vi "Launch Event Handlers.vi"(8 "error in (no error)":errorcluster, 11 "IViewable In":refnum<class "IViewable.lvclass">) -> (0 "error out":errorcluster, 3 "IViewable Out":refnum<class "IViewable.lvclass">)   [LabVIEW 2020, in "MVA Framework.lvlib" / "IViewable.lvlib" / "IViewable.lvclass"]
doc: "启动事件处理程序"
uses:
  IViewable.lvclass
  ActorEvents/IEventAggregator/IEventAggregator.lvclass
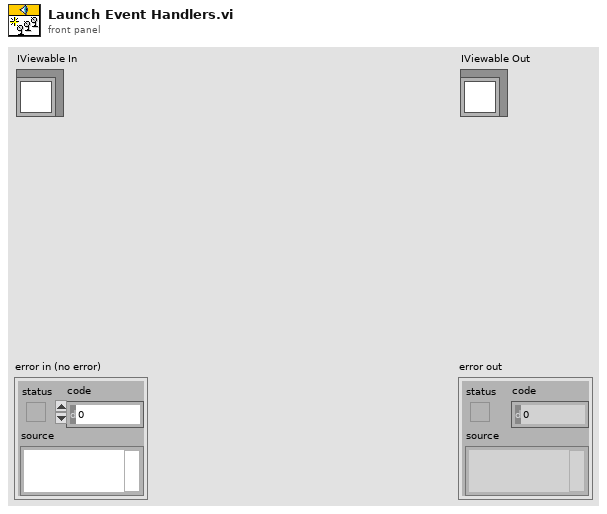
[diagram p1: front panel]
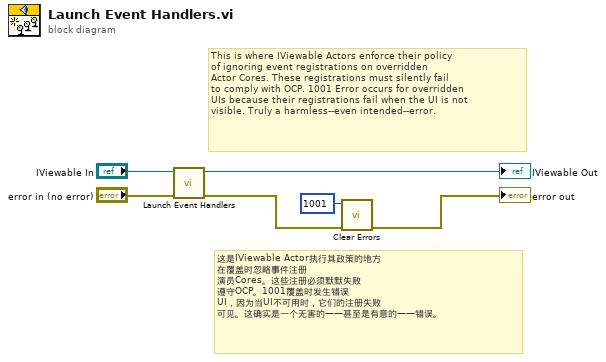
[diagram p0: block diagram]
diagram:
  # "这是IViewable Actor执行其政策的地方\n在覆盖时忽略事件注册\n演员Cores。这些注册必须默默失败\n遵守OCP。1001覆盖时发生错误\nUI，因为当UI不可用时，它们的注册失败\n可见。这确实是一个无害的——甚至是有意的——错误。"
  # "This is where IViewable Actors enforce their policy\nof ignoring event registrations on overridden\nActor Cores. These registrations must silently fail\nto comply with OCP. 1001 Error occurs for overridden\nUIs because their registrations fail when the UI is not\nvisible. Truly a harmless--even intended--error."
  n1 = call-parent "Launch Event Handlers.vi"("error in (no error)"="error in (no error)", "IEventAggregator In"="IViewable In") -> ("error out"=w4:errorcluster, "IEventAggregator Out"=→"IViewable Out":refnum<class "IViewable.lvclass">)  [unwired: 8 in]
  n2 = call <vilib>:"Clear Errors.vi"("error in (no error)"=w4, "specific error code to clear (0: all)"=1001) -> ("error out"=→"error out":errorcluster)  [unwired: 4 in, 1 out]
